vi "Obtener Path.vi"(11 "CAFE ACTOR.lvlib:CAFE ACTOR.lvclass":refnum<class "CAFE ACTOR.lvclass">) -> (3 "appended path":path)   [LabVIEW 2019, in "CAFE ACTOR.lvlib" / "CAFE ACTOR.lvclass"]
uses:
  CAFE ACTOR.lvclass
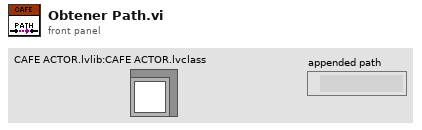
[diagram p1: front panel]
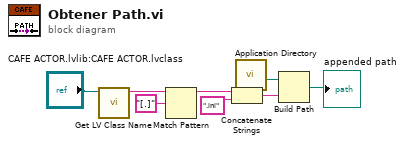
[diagram p0: block diagram]
diagram:
  n1 = call <vilib>:"Get LV Class Name.vi"("object"="CAFE ACTOR.lvlib:CAFE ACTOR.lvclass") -> ("class name"=w4:string)  [unwired: 9 in, 1 out]
  n2 = Match Pattern(string=w4, regular expression="[.]") -> (before substring=w6:string)  [unwired: 1 in, 3 out]
  n3 = Concatenate Strings(w6, ".ini" ("string")) -> (w7:string)
  n4 = call <vilib>:"Application Directory.vi"() -> ("Application Directory"=w2:path)
  n5 = Build Path(base path=w2, name or relative path=w7) -> (appended path=→"appended path":path)
